vi "Default file name.vi"() -> ()   [LabVIEW 2013]
panel:
  in  "File Base Name":string
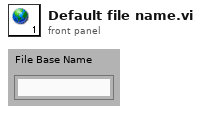
[diagram p1: front panel]
diagram:
